vi "EOL CAN_Stop CAN.vi"(8 "error in (no error)":errorcluster, 11 "XNET Session Array In":refnum<k21>[](array[refnum])) -> (0 "error out":errorcluster)   [LabVIEW 2018]
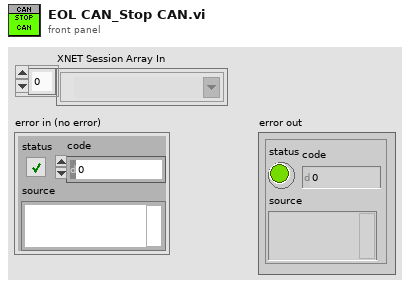
[diagram p1: front panel]
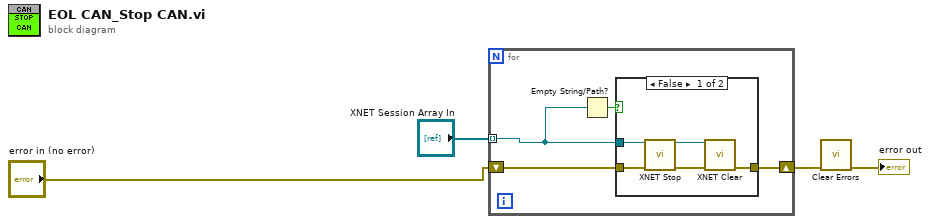
[diagram p0: block diagram]
diagram:
  n1 = for {
    shift-right: [w7] -> w2
    shift-left: "error in (no error)" -> [w8]
    tunnel: "XNET Session Array In" -> [w5] mode=indexing
    n2 = Empty String/Path?(string/path=w5) -> (empty?=w6:bool)
    n3 = case shown="False" w6 {
      tunnel: w8 -> [w11 w14]
      tunnel: [w10 w14] -> w7
      tunnel: w5 -> [w9 _]
      frame False {
        n4 = call <vilib>:"XNET Stop.vi"("session in"=w9, "error in (no error)"=w11) -> ("session out"=w12:refnum<k21>, "error out"=w13:errorcluster)  [unwired: 12 in]
        n5 = call <vilib>:"XNET Clear.vi"("session in"=w12, "error in (no error)"=w13) -> ("error out"=w10:errorcluster)  [unwired: 13 in]
      }
      frame True {
      }
    }
  }
  n6 = call <vilib>:"Clear Errors.vi"("error in (no error)"=w2) -> ("error out"=→"error out":errorcluster)  [unwired: 5 in, 1 out]
